vi "getRampAttributes.vi"(8 "error in (no error)":errorcluster, 10 "FGV Count Action":string(combo), 11 "LSR JOB Attribute":string[][](array[string])) -> (0 "error out":errorcluster, 2 "Last?":bool, 3 "subarray":string[](array[string]))   [LabVIEW 2021]
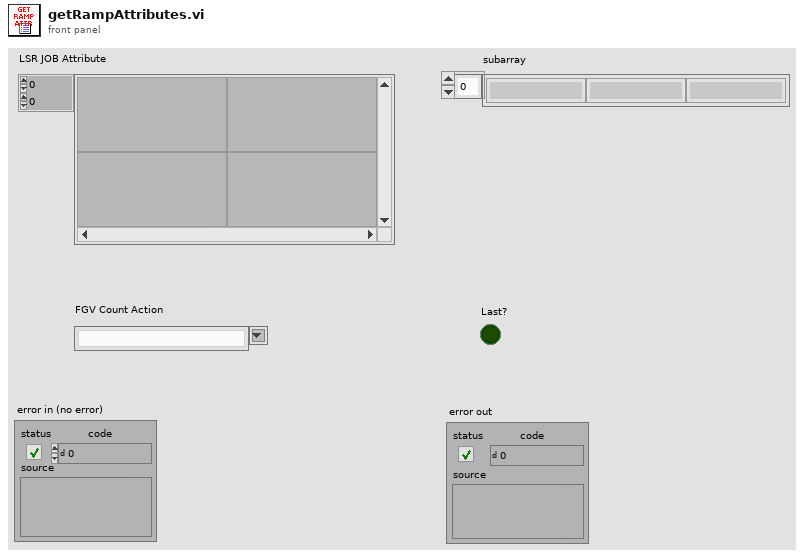
[diagram p1: front panel]
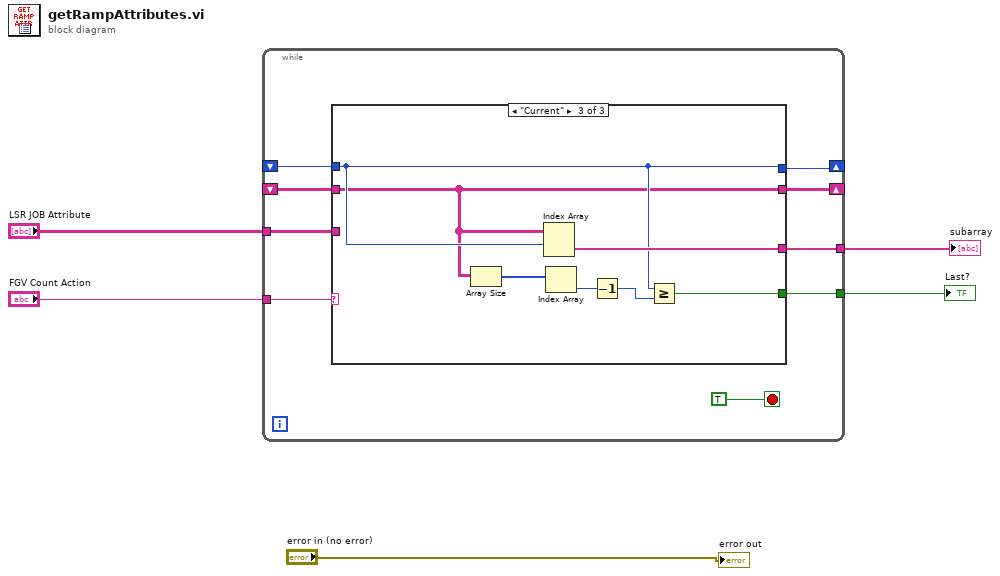
[diagram p0: block diagram]
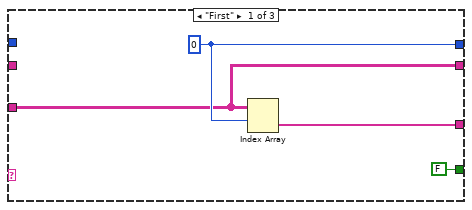
[diagram p2: hidden frame]
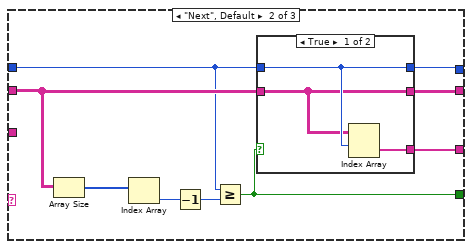
[diagram p3: hidden frame]
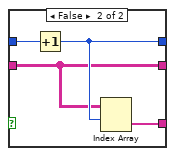
[diagram p4: hidden frame]
diagram:
  n1 = while {
    tunnel: "LSR JOB Attribute" -> [w13]
    tunnel: [w11] -> w5
    tunnel: "FGV Count Action" -> [w10]
    shift-right: [w9] -> _
    shift-left: _ -> [w12]
    tunnel: [w8] -> w3
    shift-right: [w7] -> _
    shift-left: _ -> [w6]
    stop <- TRUE ("stop") stop-if-true
    n2 = case shown="\"Current\"" w10 {
      tunnel: w13 -> [w15 _ _]
      tunnel: w12 -> [_ w21 w40]
      tunnel: [w17 w27 w41] -> w11
      tunnel: [w18 w20 w40] -> w9
      tunnel: [FALSE w22 w37] -> w8
      tunnel: [w15 w19 w35] -> w7
      tunnel: w6 -> [_ w23 w35]
      frame "First" {
        w18 = 0 ("index (row)")
        n3 = Index Array(array=w15, index (row)=w18) -> (element=w17:string[])  [unwired: 1 in]
      }
      frame "Next", Default {
        n4 = Array Size(array=w23) -> (size(s)=w26:i32[])
        n5 = Index Array(array=w26) -> (element=w25:i32)  [unwired: 1 in]
        n6 = Decrement(x=w25) -> (x-1=w24:i32)
        n7 = Greater Or Equal?(x=w21, y=w24) -> (x >= y?=w22:bool)
        n8 = case shown="True" w22 {
          tunnel: [w30 w34] -> w27
          tunnel: w23 -> [w28 w31]
          tunnel: w21 -> [w29 w33]
          tunnel: [w29 w32] -> w20
          tunnel: [w28 w31] -> w19
          frame True {
            n9 = Index Array(array=w28, index (row)=w29) -> (element=w30:string[])  [unwired: 1 in]
          }
          frame False {
            n10 = Increment(x=w33) -> (x+1=w32:i32)
            n11 = Index Array(array=w31, index (row)=w32) -> (element=w34:string[])  [unwired: 1 in]
          }
        }
      }
      frame "Current" {
        n12 = Array Size(array=w35) -> (size(s)=w39:i32[])
        n13 = Index Array(array=w35, index (row)=w40) -> (element=w41:string[])  [unwired: 1 in]
        n14 = Index Array(array=w39) -> (element=w38:i32)  [unwired: 1 in]
        n15 = Decrement(x=w38) -> (x-1=w36:i32)
        n16 = Greater Or Equal?(x=w40, y=w36) -> (x >= y?=w37:bool)
      }
    }
  }
  "subarray" <- w5
  "Last?" <- w3
  "error out" <- "error in (no error)"
